vi "Experiment header-Calculate STATS.vi"(10 "Logging queue element":T1={"Imaging Protocol"=enum."Live Imaging", "Number of Trials"=0, "Frame Size"=100, "# Averaged frames"=0, "Dwell time (us)"=0.1, "Index of Z-plane"=0, "Timelapse?"=FALSE, "Logging process is active"=FALSE, "Speed logging enabled"=FALSE, "tdms file ref"=refnum, "path"=path "", "Trial Number"=0, "Expected # points acquired"=FALSE, "Manually stopped"=FALSE, "Last trial"=FALSE, "Ch0 data"=[], "Ch1 data"=[], "Ref Data"=[], "Ref Frame Time"=[], "Image Time"=[], "Continuous Time"=[], "Ref X Length"=0, "Ref Y Length"=0, "# Ref Averaged frames"=0, "Ref Dwell time (us)"=0.0, "Points acquired"={"Ch0 last trial"=0, "Ch1 last trial"=0, "All trials"=0}, "HW Timings File"=refnum} {"Ref Dwell time (us)" format="%#.6g"; "Frame Size" items=["100X100"=100, "128X128"=128, "200X200"=200, "256X256"=256, "512X512"=512, "1024x1024"=1024, "2048x2048"=2048]; "Dwell time (us)" format="%#.6g"}, 11 "Timelapse frames saved":u32) -> (1 "Number of acquired frames":dbl, 2 "Acquisition time (ms)":dbl format="%#_9f", 3 "Total number of points acquired (Ch0)":dbl)   [LabVIEW 2017]
uses:
  Typedefs/Logging queue element.ctl
  Typedefs/Imaging Protocols enum.ctl
  Typedefs/Frame Size.ctl
  Typedefs/Acquired points count.ctl
  Typedefs/Header file interface module functions enum.ctl
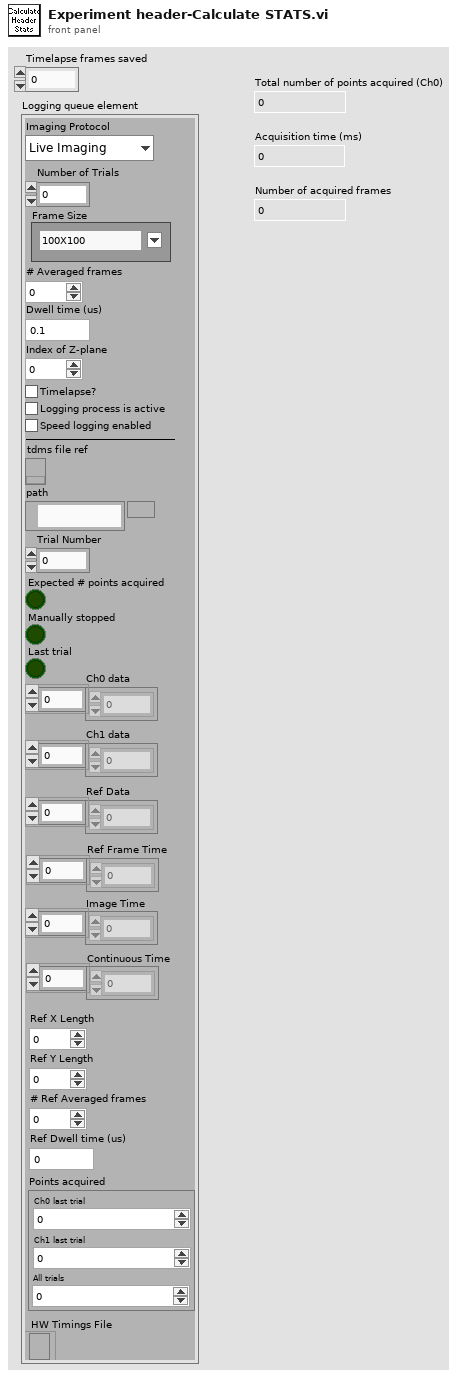
[diagram p1: front panel]
types:
  T1 = typedef "Logging queue element.ctl" = cluster{"Imaging Protocol":T2, "Number of Trials":u16, "Frame Size":T3, "# Averaged frames":u16, "Dwell time (us)":dbl, "Index of Z-plane":i32, "Timelapse?":bool, "Logging process is active":bool, "Speed logging enabled":bool, "tdms file ref":refnum<k34>, "path":path, "Trial Number":i32, "Expected # points acquired":bool, "Manually stopped":bool, "Last trial":bool, "Ch0 data":u32[], "Ch1 data":u32[], "Ref Data":u32[], "Ref Frame Time":u64[], "Image Time":u64[], "Continuous Time":u64[], "Ref X Length":u16, "Ref Y Length":u16, "# Ref Averaged frames":u16, "Ref Dwell time (us)":dbl, "Points acquired":T4, "HW Timings File":refnum<file>}
  T2 = typedef "Imaging Protocols enum.ctl" = enum16{"AOL Z-Stack", "Motor Z Stack", "Functional Acquisition", "Single Plane Acquisition", "Volume Acquisition", "Live Imaging", "Live Plane Imaging", "Live Volume Imaging"}
  T3 = typedef "Frame Size.ctl" = u16
  T4 = typedef "Acquired points count.ctl" = cluster{"Ch0 last trial":u64, "Ch1 last trial":u64, "All trials":u64}
  T5 = typedef "Header file interface module functions enum.ctl" = enum16{"Load experiment header file", "Save experiment header file", "Clear stored values", "Read stored values", "Update specific value in memory", "Update values in memory"}
  T6 = typedef "AOL_Globals.ctl" = cluster{"Imaging Protocol":T2, "Number of POI":u16, "Number of Miniscans":u16, "Number of Trials":u16, "Number of Cycles ":u64, "# Averaged Frames":u16, "Laser power (%)":u8, "Pockels (V)":dbl, "Acquisition Length (sec)":dbl, "Fill time (us)":dbl, "POI Dwell time (us)":dbl, "Miniscan Dwell time per pixel (us)":dbl, "PMT 1":dbl, "PMT 2":dbl, "Back Apperture (mA)":dbl, "Frame Size":T3, "Center Frequency":dbl, "Field of View (norm)":dbl, "DwellTime (us)":dbl, "Wavelength (nm)":dbl, "Zoom":dbl, "AOL Z":dbl, "AOL Mode":T7, "GridXY":dbl, "GridZ":dbl, "TriggerPeriod (sec)":dbl, "Number of Pixels in Miniscan":u16, "Experiment folder path":path, "X centre":dbl, "Y centre":dbl, "Angle (degrees)":dbl, "Plane Mode":T8, "Threshold":u16[], "Regenerate Chirps":bool, "Rectangle ROI length (pixels)":u16, "Rectangle ROI height (pixels)":u16, "AOD fill":u16, "StartupDelay":i32, "Samples Wait after Trigger":u16, "Slip Cycle":u32, "Add Cycle":bool, "Functional Mode":T9, "Z Start":dbl, "Z Stop":dbl, "# Planes":i32}
  T7 = typedef "AOL modes.ctl" = enum16{"Raster", "Structural", "Pointing", "Mini Scan", "Alignment"}
  T8 = typedef "Plane Mode.ctl" = u16
  T9 = typedef "Functional Mode.ctl" = enum16{"Point", "Line", "Patch", "Plane", "Volume"}
  T10 = typedef "Header parameters cluster-ALL.ctl" = cluster{"LOGIN":T11, "GLOBAL PARAMETERS":T12, "IMAGING MODES":T14, "TIME SERIES":T15, "MOTOR Z-STACK ":T17, "AOL Z-STACK":T18, "FUNCTIONAL IMAGING":T19, "VOLUME IMAGING":T19, "MOVEMENT CORRECTION":T20, "CALIBRATION":T22, "STATISTICS":T23, "BIOLOGY INFORMATION":T24}
  T11 = typedef "Header params -Login.ctl" = cluster{"User":string, "Profile":string, "Software Version":string, "Experiment Date Time":timestamp}
  T12 = typedef "Header params-Global Parameters.ctl" = cluster{"MicroscopeID":string, "Microscope Type":string, "Objective":string, "Field of View (um)":dbl, "Fill time (us)":dbl, "Experiment Type":T13, "Stimuli Trigger":bool, "Speed Logging":bool}
  T13 = typedef "Experiment Type.ctl" = enum16{"In vivo", "In vitro", "Testing", "Calibration", "Other"}
  T14 = typedef "Header params-Imaging Modes.ctl" = cluster{"Time Series":bool, "Motor Zstack":bool, "AOL Zstack":bool, "Functional Imaging":bool, "Volume Imaging":bool}
  T15 = typedef "Header params-Time Series.ctl" = cluster{"Basic Image meta data":T16, "AOL z":dbl}
  T16 = typedef "Header params-Basic image meta data.ctl" = cluster{"Wavelength (nm)":dbl, "# averaged frames":dbl, "laser power (%)":dbl, "Pockels":dbl, "pixel dwell time (us)":dbl, "pmt 1":dbl, "pmt 2":dbl, "back apperture":dbl, "zoom":dbl, "field of view":dbl, "Frame Size":T3, "AOL x centre":dbl, "AOL y centre":dbl, "Stage x position":dbl, "Stage y position":dbl, "Stage z position":dbl}
  T17 = typedef "Header params-Motor Z-stack.ctl" = cluster{"Hdr Basic Image meta data":T16, "Z Start":dbl, "Z Stop":dbl, "No of Planes":i32}
  T18 = typedef "Header params-AOL Z-stack.ctl" = cluster{"Hdr Basic Image meta data":T16, "Z Start":dbl, "Z Stop":dbl, "No of Planes":i32}
  T19 = typedef "Header params-Functional Imaging.ctl" = cluster{"Functional Mode":T9, "Pockels Modulation":bool, "Number of pois":dbl, "Number of miniscans":dbl, "Number of cycles":dbl, "Number of trials":dbl, "Miniscan dwell time per pixel (us)":dbl, "Number of pixels in miniscan":dbl, "poi dwell time":dbl, "Rectangle ROI length":dbl, "Rectangle ROI height":dbl, "AOL Mode":T7, "Plane Mode":T8, "video length (sec)":dbl, "Frame rate (fps)":dbl, "Stimuli Timing (usec)":dbl, "Acquisition Length":dbl, "Basic Image meta data":T16, "Z Start (um)":dbl, "Z Stop (um)":dbl}
  T20 = typedef "Header params-Movement correction.ctl" = cluster{"Movement Correction":bool, "Axial Reference":bool, "Reference X Pixels":dbl, "Reference Y Pixels":dbl, "Reference Source":T21, "Reference dwell time (us)":dbl, "Number of Z lines":dbl, "Size of Z pixels":dbl, "Axial Pixels":dbl, "Reference Zoom":dbl, "Reference Average":dbl, "Proportional Scale":dbl, "Integral Scale":dbl, "Proportional Scale Z":dbl, "Integral Scale Z":dbl, "Scan Interval":dbl, "Ref Plot Refresh Rate":dbl}
  T21 = typedef "Reference source.ctl" = enum16{"Green channel", "Red channel"}
  T22 = typedef "Header params-Calibration Setup.ctl" = cluster{"Pockels Calibration File":path, "Calibration_ini file":path, "Setup_ini file":path}
  T23 = typedef "Header params-statistics.ctl" = cluster{"Z-stack duration (sec)":dbl, "Number of acquired data-points":dbl, "Acquisition time (ms)":dbl, "Number of acquired frames":dbl, "Intertrial times":dbl[]}
  T24 = typedef "Biology Information.ctl" = cluster{"Animal Code or Name":string, "Animal DoB":string, "Animal Age":string, "Animal Sex":string, "Animal Weight":string, "Date of Injection":string, "Date of Implant":string, "Site of Injection":string, "Animal Ear Notch":string, "AAV constructs":string, "Genetic background":string, "Optical reporter":string, "Region of brain imaged":string, "Other \ncomments":string}
  T25 = typedef "ROI parameters data type.ctl" = cluster{"ROI index":dbl, "ROI ID":dbl, "ROI Time (ns)":dbl, "Pixels in ROI":dbl, "X start":dbl, "Y start":dbl, "Z start":dbl, "X stop":dbl, "Y stop":dbl, "Z stop":dbl, "Angle (deg)":dbl, "Composite ID":dbl, "Number of lines":dbl, "Frame Size":dbl, "Zoom":dbl, "Laser Power (%)":dbl, "ROI group ID":dbl, "Z Plane Idx":i32[], "Z Plane codes":i32[]}
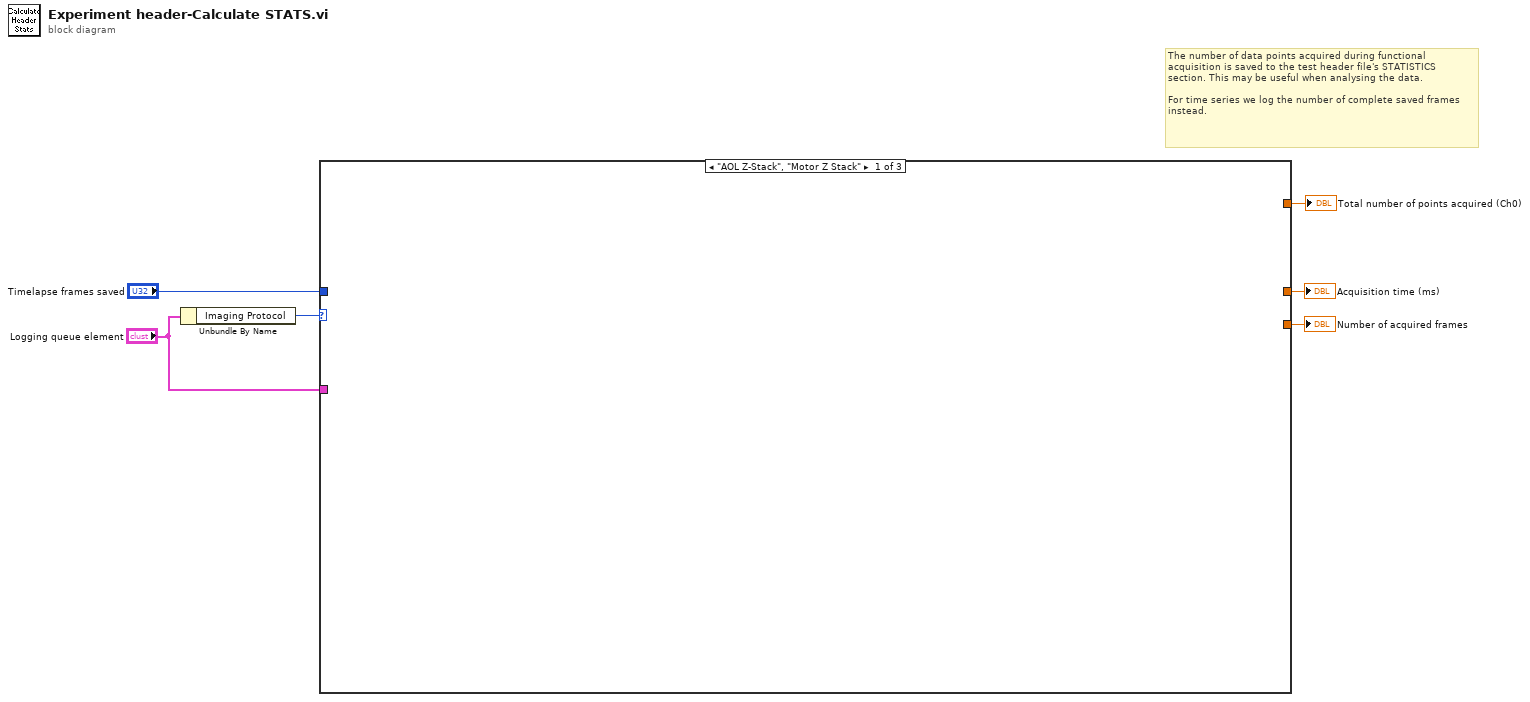
[diagram p0: block diagram]
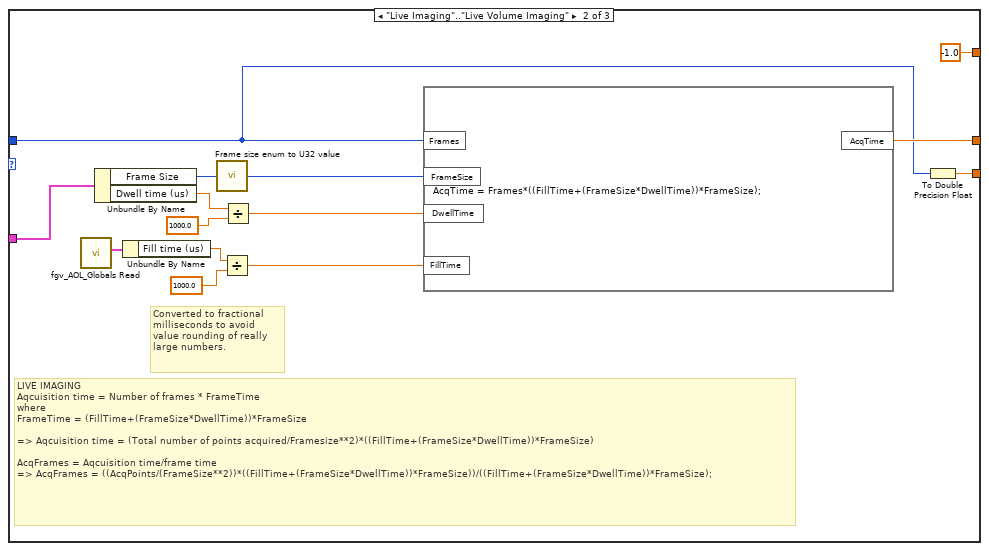
[diagram p2: hidden frame]
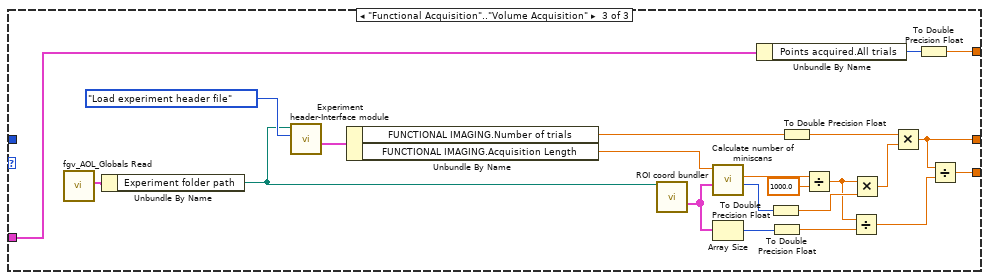
[diagram p3: hidden frame]
diagram:
  # "The number of data points acquired during functional acquisition is saved to the test header file's STATISTICS section. This may be useful when analysing the data.\n\nFor time series we log the number of complete saved frames instead."
  n1 = Unbundle By Name("Logging queue element") -> ("Imaging Protocol"=w6:T2)
  n2 = case shown="\"AOL Z-Stack\", \"Motor Z Stack\"" w6 {
    tunnel: [_ w20 w32] -> w5
    tunnel: [_ w8 w30] -> w4
    tunnel: "Logging queue element" -> [_ w10 w25]
    tunnel: [_ -1.0 ("Ch0") w24] -> w2
    tunnel: "Timelapse frames saved" -> [_ w7 _]
    frame "AOL Z-Stack", "Motor Z Stack" {
    }
    frame "Live Imaging".."Live Volume Imaging" {
      # "LIVE IMAGING\nAqcuisition time = Number of frames * FrameTime\nwhere\nFrameTime = (FillTime+(FrameSize*DwellTime))*FrameSize\n\n=> Aqcuisition time = (Total number of points acquired/Framesize**2)*((FillTime+(FrameSize*DwellTime))*FrameSize)\n\nAcqFrames = Aqcuisition time/frame time\n=> AcqFrames = ((AcqPoints/(FrameSize**2))*((FillTime+(FrameSize*DwellTime))*FrameSize))/((FillTime+(FrameSize*DwellTime))*FrameSize);"
      # "Converted to fractional milliseconds to avoid value rounding of really large numbers."
      n3 = call "fgv_AOL_Globals Read.vi"() -> ("AOL_Globals"=w15:T6)  [unwired: 9 in, 2 out]
      n4 = Unbundle By Name(w10) -> ("Frame Size"=w12:T3, "Dwell time (us)"=w11:dbl)
      n5 = Unbundle By Name(w15) -> ("Fill time (us)"=w18:dbl)
      n6 = call "Frame size enum to U32 value.vi"("Value"=w12) -> ("Frame Size U32"=w19:u32)
      n7 = Divide(x=w18, y=1000.0) -> (x/y=w14:dbl)
      n8 = Divide(x=w11, y=1000.0) -> (x/y=w13:dbl)
      n9 = formula code="AcqTime = Frames*((FillTime+(FrameSize*DwellTime))*FrameSize);"("FrameSize"=w19, "DwellTime"=w13, "FillTime"=w14, "Frames"=w7) -> ("AcqTime"=w20:dbl)
      n10 = To Double Precision Float(number=w7) -> (double precision float=w8:dbl)
    }
    frame "Functional Acquisition".."Volume Acquisition" {
      n11 = call "fgv_AOL_Globals Read.vi"() -> ("AOL_Globals"=w41:T6)  [unwired: 9 in, 2 out]
      n12 = Unbundle By Name(w41) -> ("Experiment folder path"=w22:path)
      n13 = call "Experiment header-Interface module.vi"("Function"=Header_file_interface_module_functions_enum."Load experiment header file", "Experiment data folder path"=w22) -> ("All header parameters out"=w21:T10)  [unwired: 8 in, 1 out]
      n14 = Unbundle By Name(w21) -> ("FUNCTIONAL IMAGING.Number of trials"=w35:dbl, "FUNCTIONAL IMAGING.Acquisition Length"=w42:dbl)
      n15 = call "ROI coord bundler.vi"("Experiment folder path"=w22) -> ("ROI Attributes"=w33:T25[])  [unwired: 6 in, 8 out]
      n16 = call "Calculate number of miniscans.vi"("XYZ Coordinates"=w33, "Acquisition length (sec)"=w42) -> ("Number of cycles"=w38:u64, "Cycle time (us)"=w40:dbl)  [unwired: 7 in, 1 out]
      n17 = Array Size(array=w33) -> (size(s)=w31:i32)
      n18 = Unbundle By Name(w25) -> ("Points acquired.All trials"=w26:u64)
      n19 = To Double Precision Float(number=w38) -> (double precision float=w37:dbl)
      n20 = To Double Precision Float(number=w31) -> (double precision float=w28:dbl)
      n21 = To Double Precision Float(number=w35) -> (double precision float=w34:dbl)
      n22 = Divide(x=w40, y=1000.0) -> (x/y=w29:dbl)
      n23 = Divide(x=w29, y=w28) -> (x/y=w27:dbl)
      n24 = Multiply(x=w29, y=w37) -> (x*y=w36:dbl)
      n25 = Multiply(x=w34, y=w36) -> (x*y=w32:dbl)
      n26 = To Double Precision Float(number=w26) -> (double precision float=w24:dbl)
      n27 = Divide(x=w32, y=w27) -> (x/y=w30:dbl)
    }
  }
  "Total number of points acquired (Ch0)" <- w2
  "Number of acquired frames" <- w4
  "Acquisition time (ms)" <- w5
